vi "get_images_for_sample.vi"(8 "Error In":errorcluster, 10 "Sample":string, 11 "File Path":path) -> (0 "Error Out":errorcluster, 3 "Image Names":string[](array[string]))   [LabVIEW 2019]
doc: "Returns all of the images for a given sample name in a given directory."
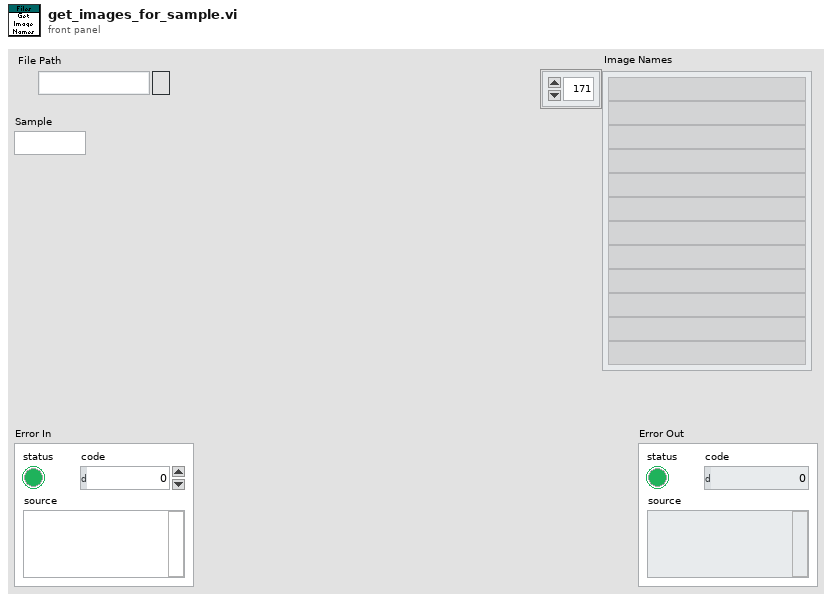
[diagram p1: front panel]
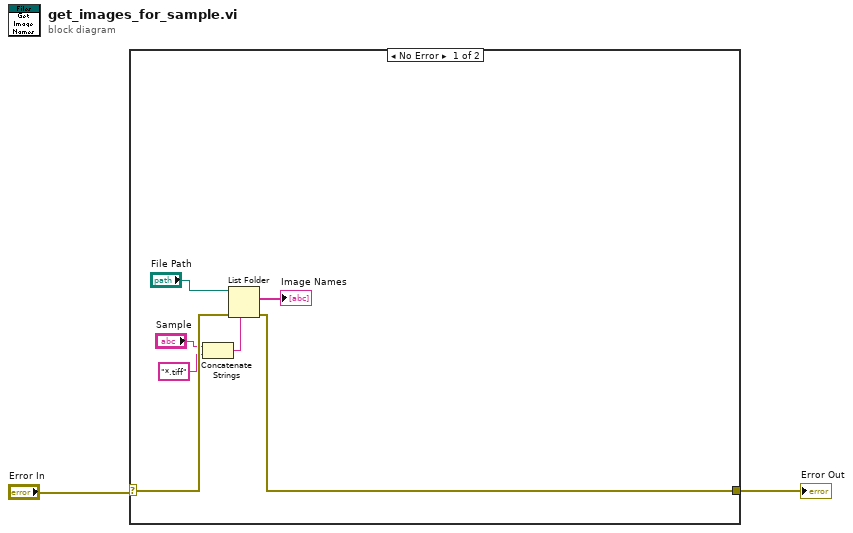
[diagram p0: block diagram]
diagram:
  n1 = case shown="No Error" "Error In" {
    selector: "Error In" -> [w8 w10]
    tunnel: [w3 w10] -> w1
    frame No Error {
      n2 = Concatenate Strings("Sample", "*.tiff" ("pattern")) -> (w5:string)
      n3 = List Folder(path="File Path", pattern=w5, error in=w8) -> (filenames=→"Image Names":string[], error out=w3:errorcluster)  [unwired: 1 in, 2 out]
    }
    frame Error {
    }
  }
  "Error Out" <- w1
